vi "MGI SZL Extract File.vi"(7 "Confirm Overwrite? (F)":bool, 8 "Error In":errorcluster, 9 "Entry Path In Zip":path=path "D:/temp/Top.zip", 10 "Target Path":path=path "D:/temp/Top.zip", 11 "Zip File":refnum<k24>) -> (0 "Error Out":errorcluster, 1 "Canceled?":bool, 3 "Zip File Out":refnum<k24>)   [LabVIEW 2020]
doc: "Extracts the entry specified by entry path in zip from the zip file to the target path. Entry path in zip should be the relative path within the zip file. If the target path already exists you can have a dialog pop up to confirm overwriting by wiring TRUE to confirm overwrite?.\n\nThis VI relies on the Sharp Zip Library which is a .NET assembly written in C# by Mike Krueger. It is licenced under the GPL with a special exception permitting independent modules to link to the library regardless of the license terms of the independent module. \n\nMore information about the library and its license is available from:\nhttp://www.icsharpcode.net/opensource/sharpziplib/\n\nAuthored by Matthew G. Harrison\nsupport@mooregoodideas.com\nwww.mooregoodideas.com\n\nCopyright (c) 2010, Moore Good Ideas, Inc.\n\nAll rights reserved.\n\nRedistribution and use in source and binary forms, with or without modification, are permitted provided that the following conditions are met:\n\n * Redistributions of source code must retain the above copyright notice, this list of conditions and the following disclaimer.\n * Redistributions in binary form must reproduce the above copyright notice, this list of conditions and the following disclaimer in the documentation and/or other materials provided with the distribution.\n * Neither the name of Moore Good Ideas, Inc. nor the names of its contributors may be used to endorse or promote products derived from this software without specific prior written permission.\n\nTHIS SOFTWARE IS PROVIDED BY THE COPYRIGHT HOLDERS AND CONTRIBUTORS \"AS IS\" AND ANY EXPRESS OR IMPLIED WARRANTIES, INCLUDING, BUT NOT LIMITED TO, THE IMPLIED WARRANTIES OF MERCHANTABILITY AND FITNESS FOR A PARTICULAR PURPOSE ARE DISCLAIMED. IN NO EVENT SHALL THE COPYRIGHT OWNER OR CONTRIBUTORS BE LIABLE FOR ANY DIRECT, INDIRECT, INCIDENTAL, SPECIAL, EXEMPLARY, OR CONSEQUENTIAL DAMAGES (INCLUDING, BUT NOT LIMITED TO, PROCUREMENT OF SUBSTITUTE GOODS OR SERVICES; LOSS OF USE, DATA, OR PROFITS; OR BUSINESS INTERRUPTION) HOWEVER CAUSED AND ON ANY THEORY OF LIABILITY, WHETHER IN CONTRACT, STRICT LIABILITY, OR TORT (INCLUDING NEGLIGENCE OR OTHERWISE) ARISING IN ANY WAY OUT OF THE USE OF THIS SOFTWARE, EVEN IF ADVISED OF THE POSSIBILITY OF SUCH DAMAGE."
uses:
  C:/Program Files/National Instruments/LabVIEW 2020/user.lib/_MGI/File/Zip/Support Files/ICSharpCode.SharpZipLib.dll
  Support Files/ICSharpCode.SharpZipLib.dll
  <userlib>/_MGI/File/MGI Create Directory Chain Behavior Enum.ctl
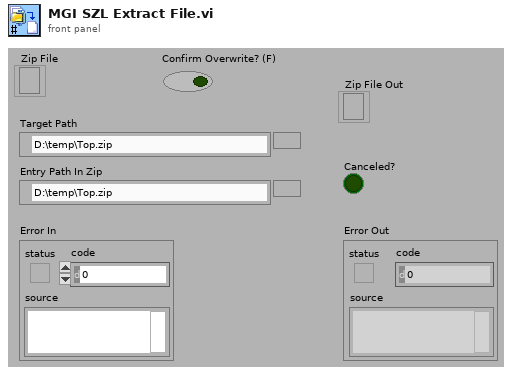
[diagram p1: front panel]
types:
  T1 = typedef "MGI Create Directory Chain Behavior Enum.ctl" = enum16{"Auto Detect", "Path Contains a File", "Path Does Not Contain a File"}
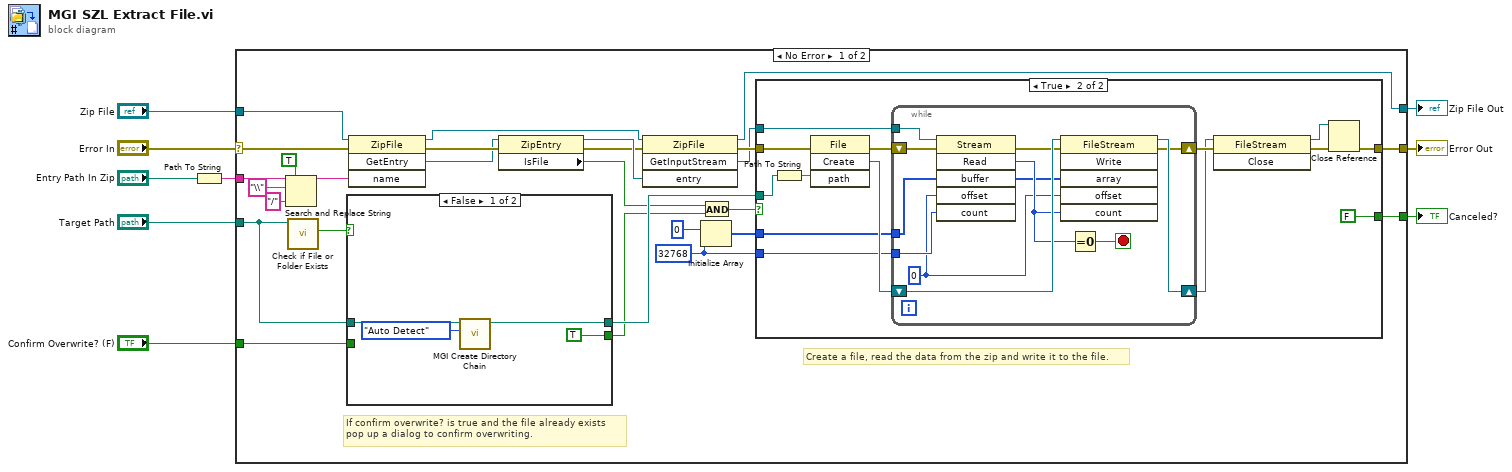
[diagram p0: block diagram]
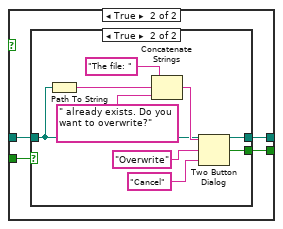
[diagram p2: hidden frame]
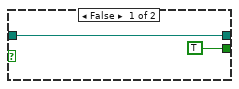
[diagram p3: hidden frame]
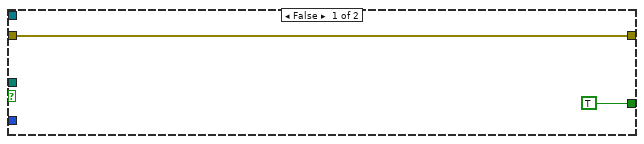
[diagram p4: hidden frame]
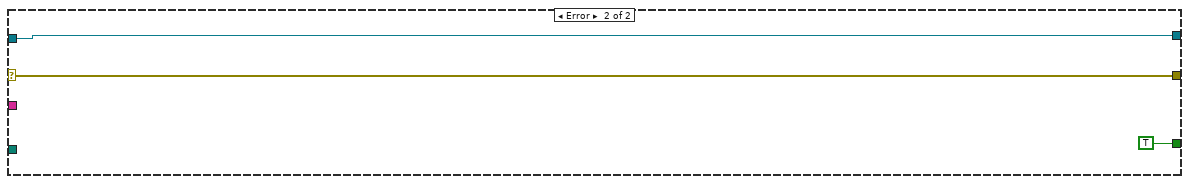
[diagram p5: hidden frame]
diagram:
  n1 = Path To String(path="Entry Path In Zip") -> (string=w3:string)
  n2 = case shown="No Error" "Error In" {
    selector: "Error In" -> [w15 w85]
    tunnel: "Zip File" -> [w36 w84]
    tunnel: [w28 w85] -> w8
    tunnel: "Target Path" -> [w11 _]
    tunnel: "Confirm Overwrite? (F)" -> [w25 _]
    tunnel: w3 -> [w19 _]
    tunnel: [w14 w84] -> w5
    tunnel: [w12 TRUE] -> w1
    frame No Error {
      w29 = 32768 ("dimension size")
      # "Create a file, read the data from the zip and write it to the file."
      # "If confirm overwrite? is true and the file already exists\npop up a dialog to confirm overwriting."
      n3 = Search and Replace String(replace all?=TRUE ("replace all? (F)"), input string=w19, search string="\\", replace string="/" ("replace string (\"\")")) -> (result string=w20:string)  [unwired: 1 in, 6 out]
      n4 = call <vilib>:"Check if File or Folder Exists.vi"("path"=w11) -> ("file or folder exists?"=w10:bool)  [unwired: 8 in, 2 out]
      n5 = case shown="False" w10 {
        tunnel: w11 -> [w39 w43]
        tunnel: [w38 w41] -> w26
        tunnel: w25 -> [_ w44]
        tunnel: [TRUE ("T button?") w42] -> w22
        frame False {
          n6 = call <userlib>:"MGI Create Directory Chain.vi"("File Presence (Auto Detect)"=MGI_Create_Directory_Chain_Behavior_Enum."Auto Detect", "Path"=w39) -> ("Duplicate Path"=w38:path)  [unwired: 8 in, 1 out]
        }
        frame True {
          n7 = case shown="True" w44 {
            tunnel: w43 -> [w45 w47]
            tunnel: [TRUE ("T button?") w48] -> w42
            tunnel: [w45 w47] -> w41
            frame False {
            }
            frame True {
              n8 = Path To String(path=w47) -> (string=w50:string)
              n9 = Concatenate Strings("The file: " ("string"), w50, " already exists. Do you want to overwrite?" ("message")) -> (w49:string)
              n10 = Two Button Dialog(message=w49, 1:"Cancel" ("F button name (\"Cancel\")"), 2:"Overwrite" ("T button name (\"OK\")")) -> (T button?=w48:bool)
            }
          }
        }
      }
      n11 = invoke class="ZipFile" method="GetEntry"(reference=w36, error in=w15, "name"=w20) -> (reference out=w13:refnum<k24>, error out=w35:errorcluster, "GetEntry"=w34:refnum<k24>)  [unwired: 1 in, 1 out]
      n12 = property class="ZipEntry"(reference=w34, error in=w35) -> (reference out=w33:refnum<k24>, error out=w21:errorcluster, "IsFile"=w23:bool)
      n13 = invoke class="ZipFile" method="GetInputStream"(reference=w13, error in=w21, "entry"=w33) -> (reference out=w14:refnum<k24>, error out=w32:errorcluster, "GetInputStream"=w27:refnum<k24>)  [unwired: 1 in, 1 out]
      n14 = Initialize Array(u8 0, w29) -> (w30:u8[])
      n15 = And(x=w23, y=w22) -> (x .and. y?=w24:bool)
      n16 = case shown="True" w24 {
        tunnel: w27 -> [_ w70]
        tunnel: [w56 w57] -> w28
        tunnel: w32 -> [w56 w67]
        tunnel: w30 -> [_ w66]
        tunnel: w29 -> [_ w65]
        tunnel: w26 -> [_ w63]
        tunnel: [TRUE FALSE] -> w12
        frame False {
        }
        frame True {
          n17 = Path To String(path=w63) -> (string=w64:string)
          n18 = invoke class="File" method="Create"(error in=w67, "path"=w64) -> (error out=w68:errorcluster, "Create"=w69:refnum<k24>)  [unwired: 2 in, 2 out]
          n19 = while {
            tunnel: w70 -> [w82]
            shift-right: [w75] -> w61
            shift-left: w68 -> [w80]
            shift-right: [w77] -> w60
            shift-left: w69 -> [w81]
            tunnel: w66 -> [w72]
            tunnel: w65 -> [w74]
            stop <- w78 stop-if-true
            w73 = 0 ("offset")
            n20 = invoke class="Stream" method="Read"(reference=w82, error in=w80, "buffer"=w72, "offset"=w73, "count"=w74) -> (error out=w76:errorcluster, "Read"=w79:i32, "buffer"=w71:u8[])  [unwired: 1 in, 3 out]
            n21 = invoke class="FileStream" method="Write"(reference=w81, error in=w76, "array"=w71, "offset"=w73, "count"=w79) -> (reference out=w77:refnum<k24>, error out=w75:errorcluster)  [unwired: 1 in, 4 out]
            n22 = Equal To 0?(x=w79) -> (x = 0?=w78:bool)
          }
          n23 = invoke class="FileStream" method="Close"(reference=w60, error in=w61) -> (reference out=w59:refnum<k24>, error out=w58:errorcluster)  [unwired: 1 in, 1 out]
          n24 = Close Reference(reference=w59, error in (no error)=w58) -> (error out=w57:errorcluster)
        }
      }
    }
    frame Error {
    }
  }
  "Error Out" <- w8
  "Zip File Out" <- w5
  "Canceled?" <- w1
